vi "back_to_default_row_color.vi"(8 "error_in":errorcluster, 10 "row":i32, 11 "listbox_reference":refnum<vi>) -> (0 "error_out":errorcluster)   [LabVIEW 2019]
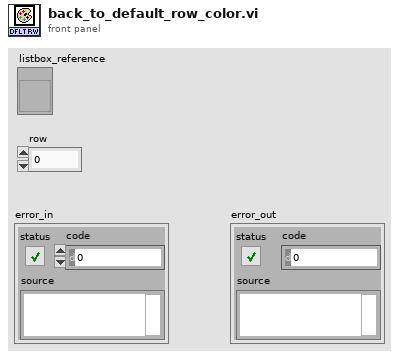
[diagram p1: front panel]
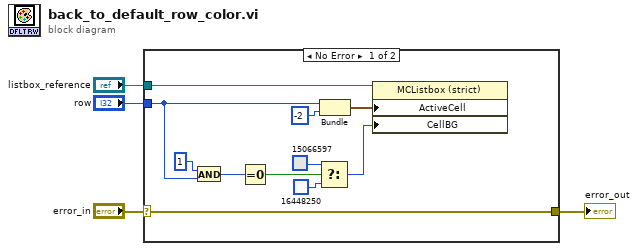
[diagram p0: block diagram]
diagram:
  n1 = case shown="No Error" "error_in" {
    selector: "error_in" -> [w7 w16]
    tunnel: "row" -> [w15 _]
    tunnel: "listbox_reference" -> [w14 _]
    tunnel: [w7 w16] -> w1
    frame No Error {
      n2 = And(x=1, y=w15) -> (x .and. y?=w11:i32)
      n3 = Equal To 0?(x=w11) -> (x = 0?=w12:bool)
      n4 = Select(t=u32 15066597, s=w12, f=u32 16448250) -> (s? t:f=w13:u32)
      n5 = Bundle("row"=w15, -2) -> (w9:cluster{"row":i32, i32})  [unwired: 1 in]
      n6 = property on="Property Node" class="MCListbox (strict)"(reference=w14, "ActiveCell"=w9, "CellBG"=w13) -> ()  [unwired: 1 in, 2 out]
    }
    frame Error {
    }
  }
  "error_out" <- w1
